vi "grascale_lvl_conv.vi"(10 "max level":dbl, 11 "Array in":dbl[](array[numeric])) -> (3 "Array out":dbl[](array[numeric]))   [LabVIEW 2020]
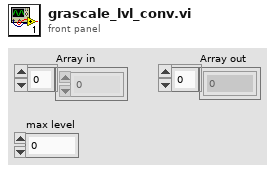
[diagram p1: front panel]
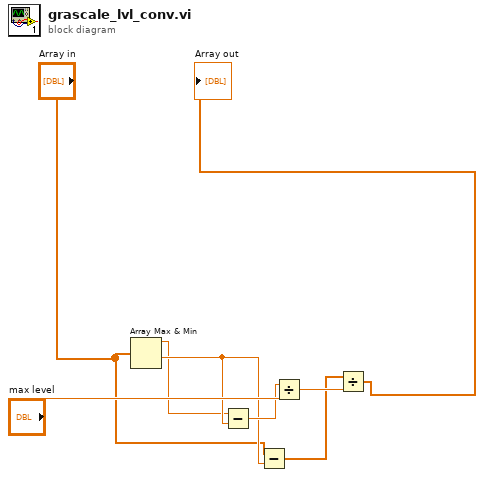
[diagram p0: block diagram]
diagram:
  n1 = Array Max & Min(array="Array in") -> (max value=w1:dbl, min value=w3:dbl)  [unwired: 2 out]
  n2 = Subtract(x=w1, y=w3) -> (x-y=w6:dbl)
  n3 = Subtract(x="Array in", y=w3) -> (x-y=w4:dbl[])
  n4 = Divide(x=w6, y="max level") -> (x/y=w8:dbl)
  n5 = Divide(x=w4, y=w8) -> (x/y=→"Array out":dbl[])
